vi "Example Pixel Matrix.vi"() -> ()   [LabVIEW 2010]
uses:
  C:/tf/play/labview/Tinkerforge.dll
  Tinkerforge.dll
panel:
  in  "uid":string="abc"
  in  "port":i32=4223
  in  "host":string="localhost"
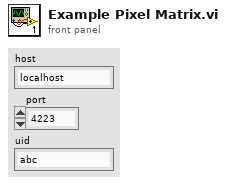
[diagram p1: front panel]
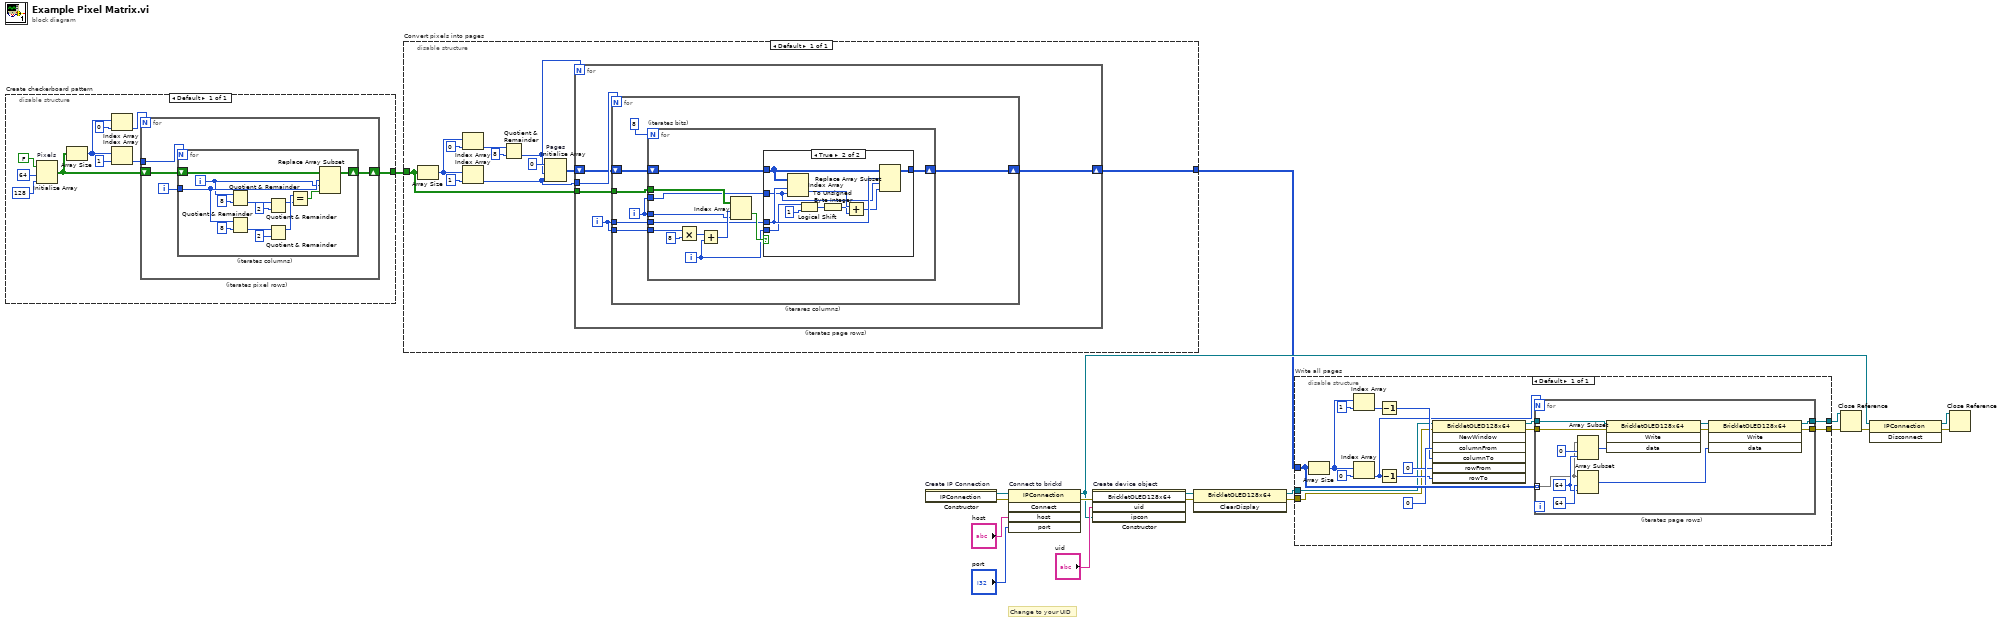
[diagram p0: block diagram]
diagram:
  # "Change to your UID"
  n1 = disable-structure "Create checkerboard pattern" shown="Default" {
    disable-tunnel: [w25] -> w6
    frame Enabled {
      n2 = Initialize Array "Pixels"(FALSE, 64 ("dimension size"), 128 ("dimension size")) -> (w24:bool[][])
      n3 = Array Size(array=w24) -> (size(s)=w21:i32[])
      n4 = Index Array(array=w21, index=0) -> (element=w20:i32)
      n5 = Index Array(array=w21, index=1) -> (element=w19:i32)
      n6 = for "(iterates pixel rows)" {
        N: w20 -> [_]
        shift-right: [w31] -> w25
        shift-left: w24 -> [w32]
        tunnel: w19 -> [w30]
        i -> [w29]
        n7 = for "(iterates columns)" {
          N: w30 -> [_]
          shift-right: [w36] -> w31
          shift-left: w32 -> [w37]
          tunnel: w29 -> [w35]
          i -> [w34]
          n8 = Quotient & Remainder(x=w34, y=8) -> (floor(x/y)=w40:i32)  [unwired: 1 out]
          n9 = Quotient & Remainder(x=w35, y=8) -> (floor(x/y)=w43:i32)  [unwired: 1 out]
          n10 = Quotient & Remainder(x=w40, y=2) -> (x-y*floor(x/y)=w38:i32)  [unwired: 1 out]
          n11 = Quotient & Remainder(x=w43, y=2) -> (x-y*floor(x/y)=w45:i32)  [unwired: 1 out]
          n12 = Equal?(x=w45, y=w38) -> (x = y?=w33:bool)
          n13 = Replace Array Subset(array=w37, new element=w33, index (row)=w35, index (col)=w34) -> (w36:bool[][])
        }
      }
    }
  }
  n14 = disable-structure "Convert pixels into pages" shown="Default" {
    disable-tunnel: w6 -> [w51]
    disable-tunnel: [w46] -> w5
    frame Enabled {
      n15 = Array Size(array=w51) -> (size(s)=w53:i32[])
      n16 = Index Array(array=w53, index=0) -> (element=w55:i32)
      n17 = Index Array(array=w53, index=1) -> (element=w48:i32)
      n18 = Quotient & Remainder(x=w55, y=8) -> (floor(x/y)=w49:i32)  [unwired: 1 out]
      n19 = Initialize Array "Pages"(u8 0, w49, w48) -> (w47:u8[][])
      n20 = for "(iterates page rows)" {
        N: w49 -> [_]
        tunnel: w48 -> [w61]
        tunnel: w51 -> [w60]
        shift-right: [w57] -> w46
        shift-left: w47 -> [w59]
        i -> [w58]
        n21 = for "(iterares columns)" {
          N: w61 -> [_]
          tunnel: w58 -> [w67]
          tunnel: w60 -> [w66]
          shift-right: [w62] -> w57
          shift-left: w59 -> [w65]
          tunnel: w58 -> [w64]
          i -> [w63]
          n22 = for "(iterates bits)" {
            N: 8 -> [_]
            tunnel: w67 -> [w80]
            tunnel: w66 -> [w76]
            tunnel: w63 -> [w75]
            shift-right: [w69] -> w62
            shift-left: w65 -> [w73]
            tunnel: w64 -> [w72]
            tunnel: w63 -> [w71]
            i -> [w70]
            n23 = Multiply(x=w80, y=8) -> (x*y=w78:i32)
            n24 = Add(x=w78, y=w70) -> (x+y=w77:i32)
            n25 = Index Array(array=w76, index (row)=w77, index (col)=w75) -> (element=w74:bool)
            n26 = case shown="True" w74 {
              tunnel: w73 -> [w81 w90]
              tunnel: w72 -> [_ w89]
              tunnel: w71 -> [_ w88]
              tunnel: w70 -> [_ w82]
              tunnel: [w81 w86] -> w69
              frame False {
              }
              frame True {
                n27 = Index Array(array=w90, index (row)=w89, index (col)=w88) -> (element=w91:u8)
                n28 = Logical Shift(y=w82, x=u8 1 ("y")) -> (x << y=w85:u8)
                n29 = To Unsigned Byte Integer(number=w85) -> (unsigned 8bit integer=w84:u8)
                n30 = Add(x=w91, y=w84) -> (x+y=w87:u8)
                n31 = Replace Array Subset(array=w90, new element=w87, index (row)=w89, index (col)=w88) -> (w86:u8[][])
              }
            }
          }
        }
      }
    }
  }
  n32 = constructor on="Create IP Connection" class="IPConnection"() -> (reference out=w18:refnum<k24>, error out=w7:errorcluster)  [unwired: 3 in, 1 out]
  n33 = invoke on="Connect to brickd" class="IPConnection" method="Connect"(reference=w18, error in=w7, "host"="host", "port"="port") -> (reference out=w9:refnum<k24>, error out=w14:errorcluster)  [unwired: 1 in, 3 out]
  n34 = constructor on="Create device object" class="BrickletOLED128x64"(error in=w14, "uid"="uid", "ipcon"=w9) -> (reference out=w12:refnum<k24>, error out=w13:errorcluster)  [unwired: 2 in, 3 out]
  n35 = invoke class="BrickletOLED128x64" method="ClearDisplay"(reference=w12, error in=w13) -> (reference out=w3:refnum<k24>, error out=w4:errorcluster)  [unwired: 1 in, 1 out]
  n36 = disable-structure "Write all pages" shown="Default" {
    disable-tunnel: w5 -> [w106]
    disable-tunnel: w4 -> [w96]
    disable-tunnel: w3 -> [w95]
    disable-tunnel: [w94] -> w1
    disable-tunnel: [w93] -> w2
    frame Enabled {
      n37 = Array Size(array=w106) -> (size(s)=w104:i32[])
      n38 = Index Array(array=w104, index=1) -> (element=w101:i32)
      n39 = Index Array(array=w104, index=0) -> (element=w92:i32)
      n40 = Decrement(x=w101) -> (x-1=w102:i32)
      n41 = Decrement(x=w92) -> (x-1=w100:i32)
      n42 = invoke class="BrickletOLED128x64" method="NewWindow"(reference=w95, error in=w96, "columnFrom"=u8 0, "columnTo"=w102, "rowFrom"=u8 0, "rowTo"=w100) -> (reference out=w97:refnum<k24>, error out=w98:errorcluster)  [unwired: 1 in, 5 out]
      n43 = for "(iterates page rows)" {
        N: w92 -> [_]
        tunnel: w106 -> [w108] mode=indexing
        tunnel: w98 -> [w119]
        tunnel: w97 -> [w118]
        tunnel: [w114] -> w94
        tunnel: [w113] -> w93
        w109 = 64 ("length")
        n44 = Array Subset(array=w108, index=0, length=w109) -> (w111:u8[])
        n45 = Array Subset(array=w108, index=64, length=w109) -> (w110:u8[])
        n46 = invoke class="BrickletOLED128x64" method="Write"(reference=w118, error in=w119, "data"=w111) -> (reference out=w116:refnum<k24>, error out=w115:errorcluster)  [unwired: 1 in, 2 out]
        n47 = invoke class="BrickletOLED128x64" method="Write"(reference=w116, error in=w115, "data"=w110) -> (reference out=w114:refnum<k24>, error out=w113:errorcluster)  [unwired: 1 in, 2 out]
      }
    }
  }
  n48 = Close Reference(reference=w1, error in (no error)=w2) -> (error out=w11:errorcluster)
  n49 = invoke class="IPConnection" method="Disconnect"(reference=w9, error in=w11) -> (reference out=w8:refnum<k24>, error out=w10:errorcluster)  [unwired: 1 in, 1 out]
  n50 = Close Reference(reference=w8, error in (no error)=w10) -> ()  [unwired: 1 out]
